vi "Handle Write Speed.vi"(6 "Time Stamp":timestamp, 8 "error in (no error)":errorcluster, 9 "Size":u64, 10 "Time":dbl, 11 "Main in":refnum<class "Main.lvclass">) -> (0 "error out":errorcluster, 3 "Main out":refnum<class "Main.lvclass">)   [LabVIEW 2025, in "Main.lvlib" / "Main.lvclass"]
uses:
  Main.lvclass
  Main.lvclass/Main.ctl
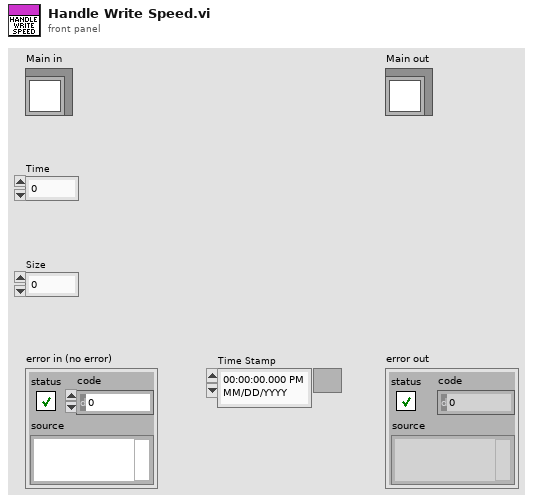
[diagram p1: front panel]
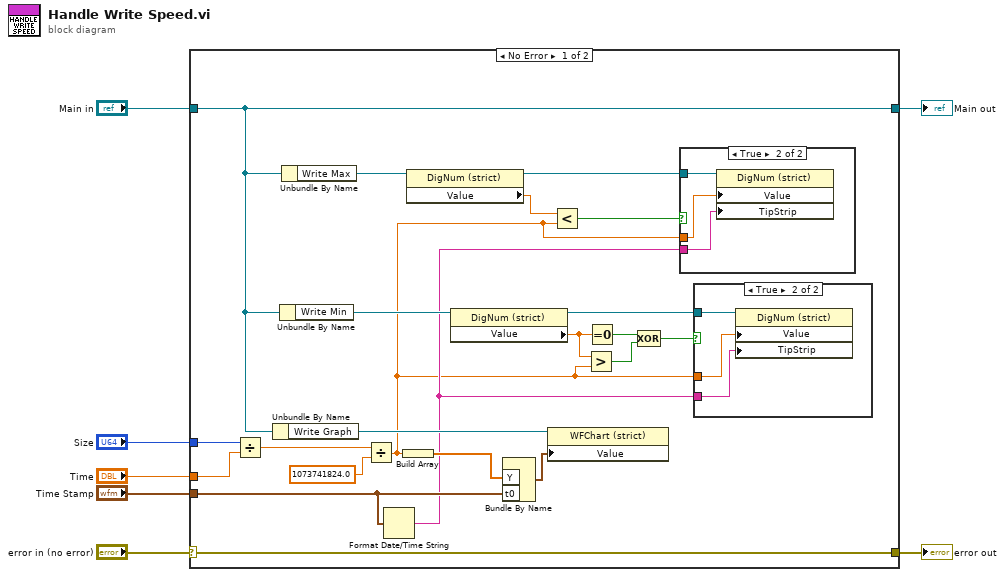
[diagram p0: block diagram]
diagram:
  n1 = case shown="No Error" "error in (no error)" {
    selector: "error in (no error)" -> [w29 w37]
    tunnel: [w29 w37] -> w2
    tunnel: [w17 w36] -> w1
    tunnel: "Main in" -> [w17 w36]
    tunnel: "Time" -> [w23 _]
    tunnel: "Size" -> [w22 _]
    tunnel: "Time Stamp" -> [w16 _]
    frame No Error {
      n2 = Divide(x=w22, y=w23) -> (x/y=w28:dbl)
      n3 = Unbundle By Name(w17) -> ("Write Graph"=w26:refnum<vi>)
      n4 = Unbundle By Name(w17) -> ("Write Min"=w18:refnum<vi>)
      n5 = Unbundle By Name(w17) -> ("Write Max"=w21:refnum<vi>)
      n6 = Divide(x=w28, y=1073741824.0 ("x")) -> (x/y=w11:dbl)
      n7 = Format Date/Time String(seconds (now)=w16) -> (date/time string=w13:string)  [unwired: 2 in]
      n8 = Build Array(w11) -> (w25:dbl[])
      n9 = property class="DigNum (strict)"(reference=w21) -> (reference out=w20:refnum<vi>, "Value"=w15:dbl)  [unwired: 1 in, 1 out]
      n10 = property class="DigNum (strict)"(reference=w18) -> (reference out=w19:refnum<vi>, "Value"=w12:dbl)  [unwired: 1 in, 1 out]
      n11 = Bundle By Name("Y"=w25, "t0"=w16) -> (w24:waveform(dbl))  [unwired: 1 in]
      n12 = property class="WFChart (strict)"(reference=w26, "Value"=w24) -> ()  [unwired: 1 in, 2 out]
      n13 = Less?(x=w15, y=w11) -> (x < y?=w14:bool)
      n14 = Greater?(x=w12, y=w11) -> (0:w8:bool)
      n15 = Equal To 0?(x=w12) -> (x = 0?=w9:bool)
      n16 = Compound Arithmetic op=XOR(w9, w8) -> (w10:bool)
      n17 = case shown="True" w14 {
        tunnel: w20 -> [_ w35]
        tunnel: w11 -> [_ w34]
        tunnel: w13 -> [_ w33]
        frame False {
        }
        frame True {
          n18 = property class="DigNum (strict)"(reference=w35, "Value"=w34, "TipStrip"=w33) -> ()  [unwired: 1 in, 2 out]
        }
      }
      n19 = case shown="True" w10 {
        tunnel: w19 -> [_ w32]
        tunnel: w11 -> [_ w31]
        tunnel: w13 -> [_ w30]
        frame False {
        }
        frame True {
          n20 = property class="DigNum (strict)"(reference=w32, "Value"=w31, "TipStrip"=w30) -> ()  [unwired: 1 in, 2 out]
        }
      }
    }
    frame Error {
    }
  }
  "error out" <- w2
  "Main out" <- w1
